vi "module-09-analog-transfer.vi"() -> ()   [LabVIEW 2019]
uses:
  <vilib>/Rock Robotics/WPI/ThirdParty/JAS_Junk/TrajLib/SlewRateLimiter_Execute.vi
  samples-common-library/Ctrl_Training_Library_Protected/CtrlTrainingLibary_Protected.lvlib
panel:
  in  "Tab Control":enum32{"Execution", "Logic"}(tab)
  out "Input 2":dbl
  out "Input 1":dbl
  out "Output":dbl
  in  "Rate 1":dbl=10.0
  in  "Input 1":dbl(slide)=10.0 scale=-100.0..100.0
  in  "Select":bool
  in  "Input 2":dbl(slide)=10.0 scale=-100.0..100.0
  in  "Rate 2":dbl=10.0
  out "Transfer":cluster{dbl, dbl, "Value_Output":dbl}(graph)
  out "Boolean 2":bool
  out "Boolean 1":bool
  # "Analog Value \nTransfer Test"
  # "Selected"
  # "Rates provide bumpless\ntransfer between values"
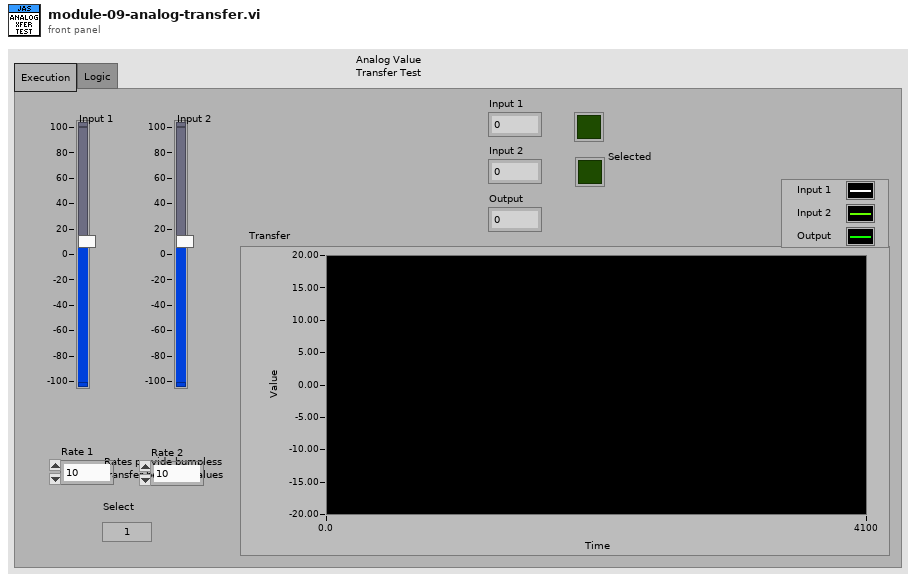
[diagram p1: front panel]
types:
  T1 = cluster{"Input 1":dbl, "Input 2":dbl, "Output":dbl}
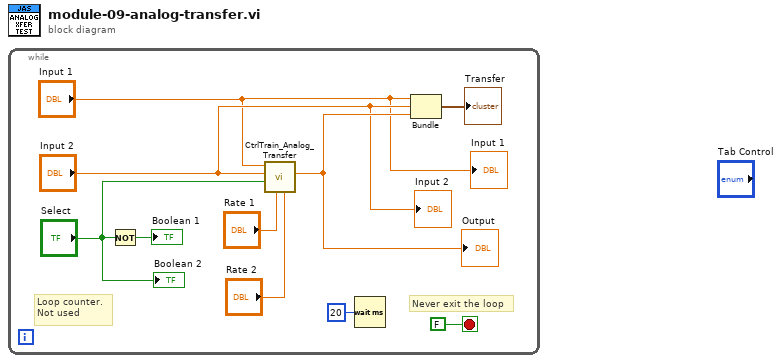
[diagram p0: block diagram]
diagram:
  n1 = while {
    stop <- FALSE stop-if-true
    # "Loop counter.\nNot used"
    # "Never exit the loop"
    n2 = Not(x="Select") -> (.not. x?=→"Boolean 1":bool)
    n3 = call "CtrlTrain_Analog_Transfer.vi"("Rate 2"="Rate 2", "Rate 1"="Rate 1", "Select 2"="Select", "Input 2"="Input 2", "Input 1"="Input 1") -> ("Output"=w6:dbl)  [unwired: 6 in]
    "Output" <- w6
    n4 = Wait (ms)(milliseconds to wait=u32 20) -> ()  [unwired: 1 out]
    n5 = Bundle("Input 1"="Input 1", "Input 2"="Input 2", "Output"=w6) -> (→"Transfer":T1)  [unwired: 1 in]
    "Input 1" <- "Input 1"
    "Input 2" <- "Input 2"
    "Boolean 2" <- "Select"
  }
